vi "createMissionWaypoints.vi"(8 "error in (no error)":errorcluster, 11 "StationKeeping in":refnum<class "StationKeeping.lvclass">) -> (0 "error out":errorcluster, 3 "StationKeeping out":refnum<class "StationKeeping.lvclass">)   [LabVIEW 2011, in "StationKeeping.lvclass"]
doc: "Using \"Station_keeping_waypoints.vi\", this VI adds the first two waypoints to the waypoint array. Rather than add more than that, it keeps a small number stored, so that the current wind can be taken into account for the pattern.\nNo sail zones are added to the second waypoint only, since the boat should be in the station at this time."
uses:
  StationKeeping.lvclass
  StationKeeping.lvclass/StationKeeping.ctl
  2 Globals/2 Global.vi
  Waypoint/Waypoint.lvclass
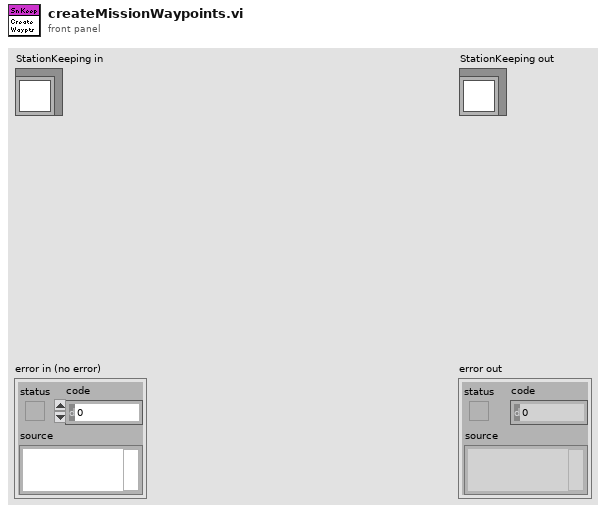
[diagram p1: front panel]
types:
  T1 = typedef "UTM Location.ctl" = cluster{"UTM Zone":dbl, "Hemisphere":enum16{"North", "South"}, "East":dbl, "North":dbl}
  T2 = typedef "UTM Circle.ctl" = cluster{"UTM Zone":dbl, "Hemisphere":enum16{"North", "South"}, "East":dbl, "North":dbl, "Radius":dbl}
  T3 = typedef "Waypoints List.ctl" = refnum<class "Waypoint.lvclass">[]
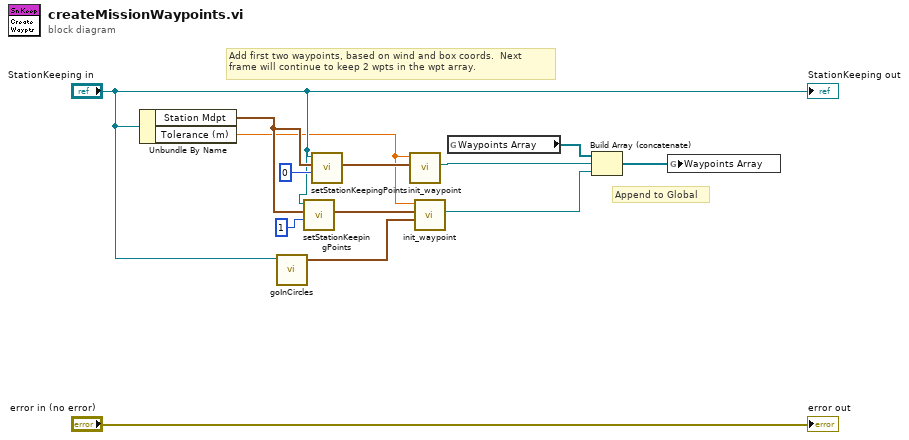
[diagram p0: block diagram]
diagram:
  # "Append to Global"
  # "Add first two waypoints, based on wind and box coords.  Next\nframe will continue to keep 2 wpts in the wpt array."
  n1 = Unbundle By Name("StationKeeping in") -> ("Station Mdpt"=w3:T1, "Tolerance (m)"=w1:dbl)
  n2 = call "goInCircles.vi"("StationKeeping in"="StationKeeping in") -> ("No Sail Circles"=w10:T2[])  [unwired: 8 in, 2 out]
  n3 = call "setStationKeepingPoints.vi"("Which Point?"=1, "Midpoint"=w3, "StationKeeping.lvclass"="StationKeeping in") -> ("Waypoint"=w9:T1)  [unwired: 8 in]
  n4 = call "setStationKeepingPoints.vi"("Which Point?"=0, "Midpoint"=w3, "StationKeeping.lvclass"="StationKeeping in") -> ("Waypoint"=w8:T1)  [unwired: 8 in]
  n5 = call "init_waypoint.vi"("Coords"=w8, "Tolerance (m)"=w1) -> ("Waypoint Out"=w12:refnum<class "Waypoint.lvclass">)  [unwired: 9 in]
  n6 = call "init_waypoint.vi"("No Sail Circles"=w10, "Coords"=w9, "Tolerance (m)"=w1) -> ("Waypoint Out"=w11:refnum<class "Waypoint.lvclass">)  [unwired: 8 in]
  n7 = global read "2 Global.vi" "Waypoints Array"() -> (w13:T3)
  n8 = Build Array (concatenate)(w13, w12, w11) -> (w5:T3)
  n9 = global write "2 Global.vi" "Waypoints Array"(w5) -> ()
  "error out" <- "error in (no error)"
  "StationKeeping out" <- "StationKeeping in"
